vi "GetVersion.vi"() -> (0 "number":i32)   [LabVIEW 2013]
panel:
  in  "Exe Path (Calling App)":path
  out "Path Out":path
  out "FileVersionInfo Out":T1
  out "File Version Info":string
  out "error out":errorcluster
  in  "error in (no error)":errorcluster
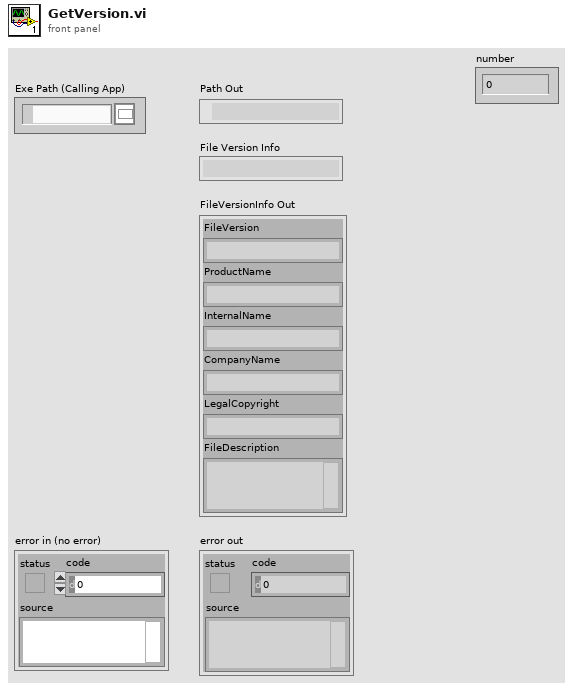
[diagram p1: front panel]
types:
  T1 = cluster{"FileVersion":string, "ProductName":string, "InternalName":string, "CompanyName":string, "LegalCopyright":string, "FileDescription":string}
  T2 = enum16{"CharacterArray", "FixedFileInfoCluster", "LanguageCode"}
  T3 = cluster{"[0]":string, "[1]":string, "[2]":string, "[3]":string, "[4]":string, "[5]":string}
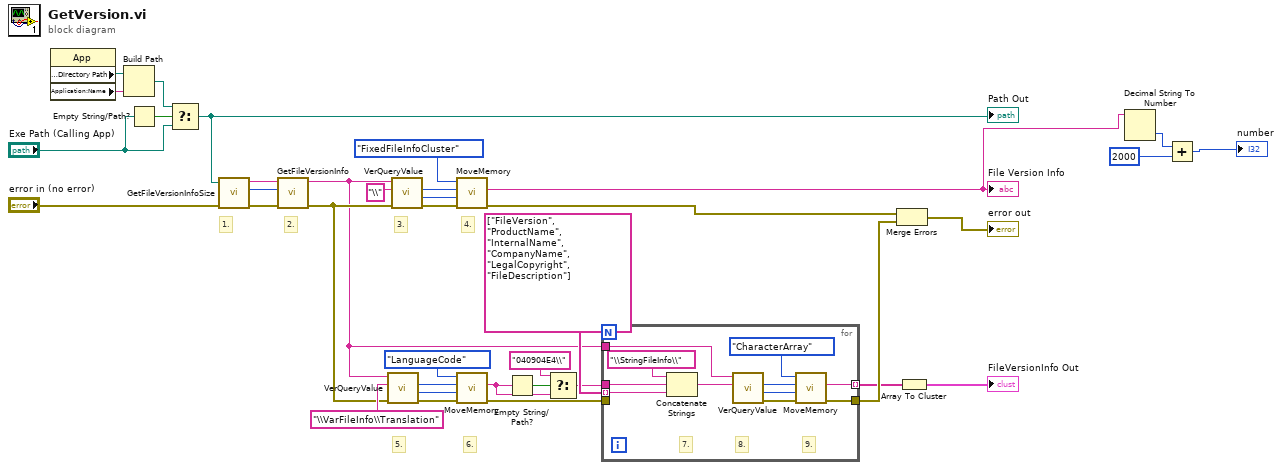
[diagram p0: block diagram]
diagram:
  # "6."
  # "4."
  # "5."
  # "3."
  # "2."
  # "1."
  n1 = property class="App"() -> ("Application:Directory Path"=w19:path, "Application:Name"=w18:string)  [unwired: 2 in, 2 out]
  n2 = Build Path(base path=w19, name or relative path=w18) -> (appended path=w16:path)
  n3 = Empty String/Path?(string/path="Exe Path (Calling App)") -> (empty?=w17:bool)
  n4 = Select(t=w16, s=w17, f="Exe Path (Calling App)") -> (s? t:f=w14:path)
  "Path Out" <- w14
  n5 = call <vilib>:"GetFileVersionInfoSize.vi"("error in (no error)"="error in (no error)", "Path"=w14) -> ("error out"=w22:errorcluster, "Size"=w21:i32, "lptstrFilename"=w23:string)  [unwired: 7 in]
  n6 = call <vilib>:"GetFileVersionInfo.vi"("error in"=w22, "Size"=w21, "lptstrFilename"=w23) -> ("error out"=w25:errorcluster, "lpData"=w9:string)  [unwired: 7 in]
  n7 = call <vilib>:"VerQueryValue.vi"("error in (no error)"=w25, "lpSubBlock"="\\VarFileInfo\\Translation", "lpData"=w9) -> ("error out"=w26:errorcluster, "puLen"=w28:u32, "lplpBuffer"=w27:u64)  [unwired: 6 in]
  n8 = call <vilib>:"VerQueryValue.vi"("error in (no error)"=w25, "lpSubBlock"="\\", "lpData"=w9) -> ("error out"=w35:errorcluster, "puLen"=w32:u32, "lplpBuffer"=w33:u64)  [unwired: 6 in]
  n9 = call <vilib>:"MoveMemory.vi"("error in (no error)"=w35, "puLen"=w32, "lplpBuffer"=w33, "Datatype"=T2."FixedFileInfoCluster") -> ("error out"=w12:errorcluster, "data"=w4:string)  [unwired: 6 in]
  "File Version Info" <- w4
  n10 = call <vilib>:"MoveMemory.vi"("error in (no error)"=w26, "puLen"=w28, "lplpBuffer"=w27, "Datatype"=T2."LanguageCode") -> ("error out"=w24:errorcluster, "data"=w7:string)  [unwired: 6 in]
  n11 = Empty String/Path?(string/path=w7) -> (empty?=w8:bool)
  n12 = Select(t="040904E4\\", s=w8, f=w7) -> (s? t:f=w5:string)
  n13 = for {
    tunnel: w9 -> [w45]
    tunnel: string[] ["FileVersion", "ProductName", "InternalName", "CompanyName", "LegalCopyright", "FileDescription"] -> [w47] mode=indexing
    tunnel: w24 -> [_]
    tunnel: [w40] -> w13
    tunnel: [w39] -> w11 mode=indexing
    tunnel: w5 -> [w38]
    # "7."
    # "9."
    # "8."
    n14 = Concatenate Strings("\\StringFileInfo\\" ("lpSubBlock"), w38, w47) -> (w46:string)
    n15 = call <vilib>:"VerQueryValue.vi"("lpSubBlock"=w46, "lpData"=w45) -> ("error out"=w43:errorcluster, "puLen"=w41:u32, "lplpBuffer"=w42:u64)  [unwired: 7 in]
    n16 = call <vilib>:"MoveMemory.vi"("error in (no error)"=w43, "puLen"=w41, "lplpBuffer"=w42, "Datatype"=T2."CharacterArray") -> ("error out"=w40:errorcluster, "data"=w39:string)  [unwired: 6 in]
  }
  n17 = Merge Errors(w12, w13) -> (→"error out":errorcluster)
  n18 = Array To Cluster(array=w11) -> (cluster=→"FileVersionInfo Out":T3)
  n19 = Decimal String To Number(string=w4) -> (number=w3:i32)  [unwired: 2 in, 1 out]
  n20 = Add(x=w3, y=2000) -> (x+y=→"number":i32)
